vi "Query_String.vi"(8 "error in":errorcluster, 11 "Query Pairs":cluster{"Field":string, "Value":string}[](array[cluster])) -> (0 "error out":errorcluster, 3 "Query String":string)   [LabVIEW 2016]
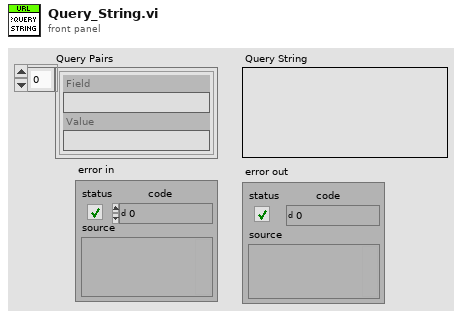
[diagram p1: front panel]
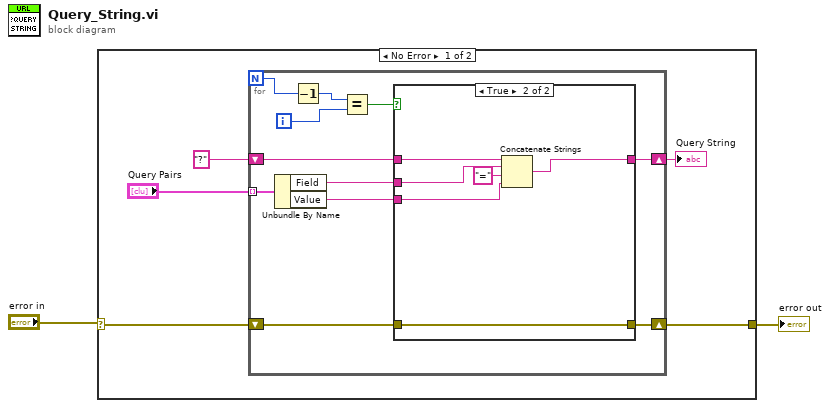
[diagram p0: block diagram]
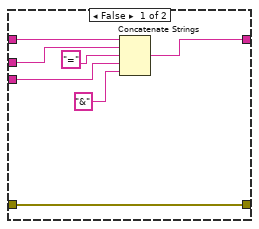
[diagram p2: hidden frame]
diagram:
  n1 = case shown="No Error" "error in" {
    selector: "error in" -> [w4 w32]
    tunnel: [w3 w32] -> w1
    frame No Error {
      n2 = for {
        N -> [w17]
        tunnel: "Query Pairs" -> [w18] mode=indexing
        shift-right: [w10] -> w5
        shift-left: "?" -> [w11]
        shift-right: [w8] -> w3
        shift-left: w4 -> [w9]
        i -> [w15]
        n3 = Unbundle By Name(w18) -> ("Field"=w13:string, "Value"=w12:string)
        n4 = Decrement(x=w17) -> (x-1=w16:i32)
        n5 = Equal?(x=w16, y=w15) -> (x = y?=w14:bool)
        n6 = case shown="True" w14 {
          tunnel: w13 -> [w24 w30]
          tunnel: w12 -> [w22 w28]
          tunnel: w11 -> [w25 w31]
          tunnel: [w20 w27] -> w10
          tunnel: w9 -> [w19 w26]
          tunnel: [w19 w26] -> w8
          frame False {
            n7 = Concatenate Strings(w25, w24, "=" ("string"), w22, "&" ("string")) -> (w20:string)
          }
          frame True {
            n8 = Concatenate Strings(w31, w30, "=" ("string"), w28) -> (w27:string)
          }
        }
      }
      "Query String" <- w5
    }
    frame Error {
    }
  }
  "error out" <- w1
